vi "呈现图片.vi"(8 "error in (no error)":errorcluster caption="错误输入（无错误）", 11 "三角形 输入":refnum<class "三角形.lvclass"> caption="DNL_LabVIEW Object in") -> (0 "error out":errorcluster caption="错误输出", 2 "Picture":picture caption="图片", 3 "三角形 输出":refnum<class "三角形.lvclass"> caption="DNL_LabVIEW Object out")   [LabVIEW 2011, in "三角形.lvclass"]
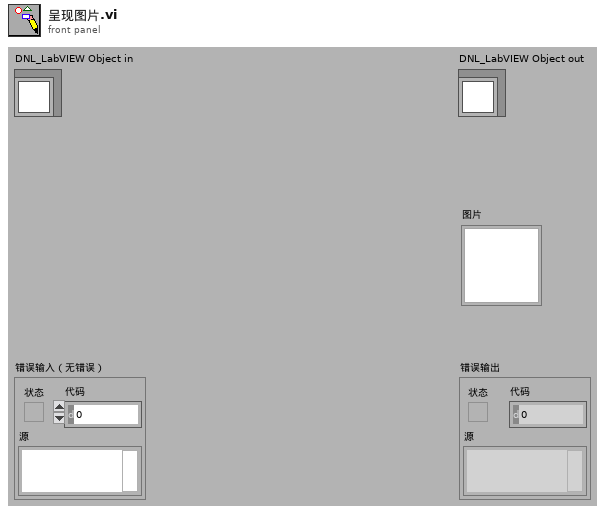
[diagram p1: front panel]
types:
  T1 = typedef "LVPointDoubleTypeDef.ctl" = cluster{"X":dbl, "Y":dbl}
  T2 = cluster{"Width":u16, "Style":enum32{"Solid", "Dash", "Dot", "DashDot", "DashDotDot"}}
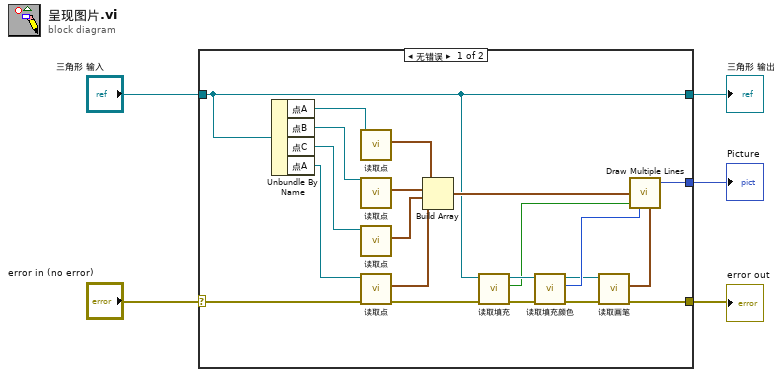
[diagram p0: block diagram]
diagram:
  n1 = case shown="无错误" "error in (no error)" {
    selector: "error in (no error)" -> [w16 w28]
    tunnel: [w8 w28] -> w4
    tunnel: "三角形 输入" -> [w12 w27]
    tunnel: [w12 w27] -> w2
    tunnel: [w17 _] -> w1
    frame No Error {
      n2 = Unbundle By Name(w12) -> ("点A"=w26:refnum<class "点.lvclass">, "点B"=w25:refnum<class "点.lvclass">, "点C"=w24:refnum<class "点.lvclass">, "点A"=w23:refnum<class "点.lvclass">)
      n3 = call "读取点.vi"("点输入"=w26) -> ("点"=w22:T1)  [unwired: 8 in, 2 out]
      n4 = call "读取点.vi"("点输入"=w25) -> ("点"=w21:T1)  [unwired: 8 in, 2 out]
      n5 = call "读取点.vi"("点输入"=w24) -> ("点"=w20:T1)  [unwired: 8 in, 2 out]
      n6 = call "读取点.vi"("error in (no error)"=w16, "点输入"=w23) -> ("error out"=w14:errorcluster, "点"=w19:T1)  [unwired: 7 in, 1 out]
      n7 = Build Array(w22, w21, w20, w19) -> (w18:T1[])
      n8 = call "读取填充.vi"("error in (no error)"=w14, "图形输入"=w12) -> ("error out"=w13:errorcluster, "填充"=w10:bool, "图形输出"=w11:refnum<class "三角形.lvclass">)  [unwired: 7 in]
      n9 = call "读取填充颜色.vi"("error in (no error)"=w13, "图形输入"=w11) -> ("error out"=w9:errorcluster, "填充颜色"=w15:u32, "图形输出"=w7:refnum<class "三角形.lvclass">)  [unwired: 7 in]
      n10 = call "读取画笔.vi"("error in (no error)"=w9, "图形输入"=w7) -> ("error out"=w8:errorcluster, "画笔"=w6:T2)  [unwired: 7 in, 1 out]
      n11 = call <vilib>:"Draw Multiple Lines.vi"("line endpoints"=w18, "fill?(F)"=w10, "color(black)"=w15, "pen"=w6) -> ("new picture"=w17:picture)  [unwired: 5 in]
    }
    frame Error {
    }
  }
  "error out" <- w4
  "三角形 输出" <- w2
  "Picture" <- w1
